vi "Try Unsigned Integer Value.vi"(8 "error in (no error)":errorcluster, 10 "Scaling Info":T1={"Bit Offset"=0, "Bit Count"=0, "LSB Resolution"=0.1, "2's Complement"=FALSE, "Big Endian"=FALSE, "Sign Bit"=FALSE}, 11 "Random Attempts":i32=100) -> (0 "error out":errorcluster)   [LabVIEW 2020, in "Unit Tests.lvlib" / "Data Scaling.lvclass"]
uses:
  Data Scaling.lvclass
  Frames & Messages/TypeDefs/Scaling Information.ctl
  <vilib>/addons/_JKI Toolkits/Caraya/classes/Assert/Assert.lvclass
  BCI-1553 API.lvlib
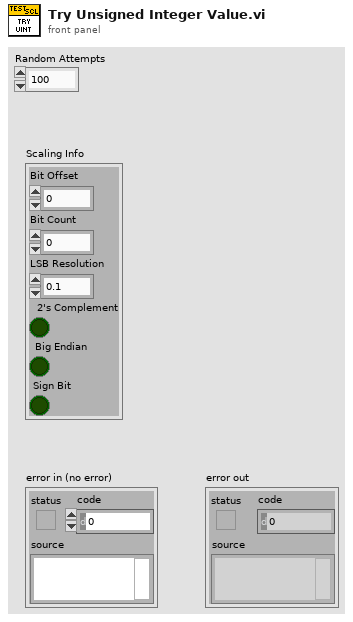
[diagram p1: front panel]
types:
  T1 = typedef "BCI-1553 API.lvlib/Scaling Information.ctl" = cluster{"Bit Offset":i32, "Bit Count":i32, "LSB Resolution":dbl, "2's Complement":bool, "Big Endian":bool, "Sign Bit":bool}
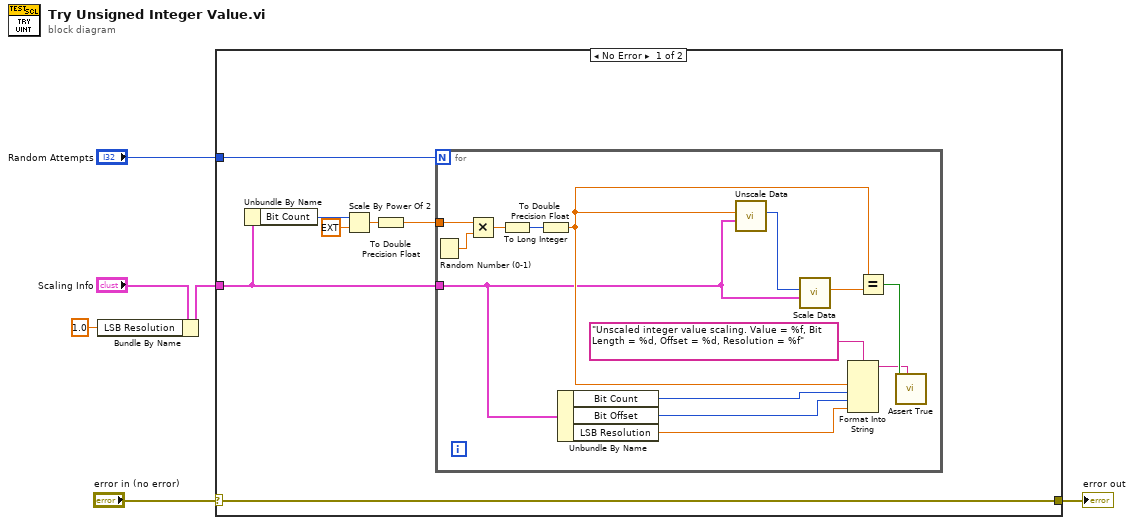
[diagram p0: block diagram]
diagram:
  n1 = Bundle By Name(cluster="Scaling Info", "LSB Resolution"=1.0) -> (w2:T1)
  n2 = case shown="No Error" "error in (no error)" {
    selector: "error in (no error)" -> [w13 w28]
    tunnel: [w13 w28] -> w5
    tunnel: "Random Attempts" -> [w12 _]
    tunnel: w2 -> [w11 _]
    frame No Error {
      n3 = Unbundle By Name(w11) -> ("Bit Count"=w10:i32)
      n4 = Scale By Power Of 2(n=w10, x=ext 1.0) -> (x*2^n=w8:ext)
      n5 = To Double Precision Float(number=w8) -> (double precision float=w7:dbl)
      n6 = for {
        N: w12 -> [_]
        tunnel: w11 -> [w17]
        tunnel: w7 -> [w18]
        n7 = Random Number (0-1)() -> (number: 0 to 1=w24:dbl)
        n8 = Multiply(x=w18, y=w24) -> (x*y=w23:dbl)
        n9 = To Long Integer(number=w23) -> (32bit integer=w22:i32)
        n10 = To Double Precision Float(number=w22) -> (double precision float=w19:dbl)
        n11 = Unbundle By Name(w17) -> ("Bit Count"=w16:i32, "Bit Offset"=w15:i32, "LSB Resolution"=w14:dbl)
        n12 = call "Unscale Data.vi"("Scaling Info"=w17, "Scaled Value"=w19) -> ("Raw Value"=w27:u64)  [unwired: 8 in, 1 out]
        n13 = call "Scale Data.vi"("Scaling Info"=w17, "Raw Value"=w27) -> ("Scaled Value"=w26:dbl)  [unwired: 8 in, 1 out]
        n14 = Format Into String(format string="Unscaled integer value scaling. Value = %f, Bit Length = %d, Offset = %d, Resolution = %f" ("Label"), w19, w16, w15, w14) -> (resulting string=w20:string)  [unwired: 2 in, 1 out]
        n15 = Equal?(x=w19, y=w26) -> (x = y?=w25:bool)
        n16 = call <vilib>:"Assert True.vi"("Label"=w20, "True?"=w25) -> ()  [unwired: 8 in, 2 out]
      }
    }
    frame Error {
    }
  }
  "error out" <- w5
